vi "Processing Loop.vi"(8 "error in":errorcluster, 11 "Queue in":refnum<queue>) -> (0 "error out":errorcluster)   [LabVIEW 2013, in "LVTM.lvlib"]
uses:
  LVTM.lvlib
  Controls_LVTM/SharedDataDVR.ctl
  Plugin/LVTM_Plugin.lvclass
  Controls_LVTM/LVTM_Config_Info.ctl
  Controls_LVTM/View.ctl
  TCP_Server/TCP_Server.lvclass
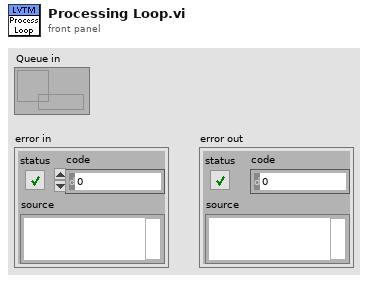
[diagram p1: front panel]
types:
  T1 = typedef "LVTM.lvlib/LVTM_Config_Info.ctl" = cluster{"Data Tree Ref":refnum<vi>, "FP Ref":refnum<vi>, "Column Data Type":enum16{"String", "Numeric"}[], "Search Clones Up To":i32, "SortOptions":cluster{"Col.pri":i32, "RevDir.pri":bool, "Col.sec":i32, "RevDir.sec":bool}, "Group/Flat (0:group)":bool, "CollapsedNodes":string[], "Show/Hide Cols":bool[], "Filtered Paths":path[], "View":T2, "File Extension Filters":string[], "Filter Global VIs":bool, "Shared":refnum<data-value>, "Active Filters":refnum<vi>, "Refresh Rate (ms)":i32, "App Instance Ring Ref":refnum<vi>, "Processing Q":refnum<queue>, "VI Ref":refnum<vi>}
  T2 = typedef "LVTM.lvlib/View.ctl" = enum16{"Group By Library", "Group By Folder", "Flat List"}
  T3 = cluster{"Shared":refnum<data-value>, "Plugins":refnum<class "LVTM_Plugin.lvclass">[], "UIConfig":T1}
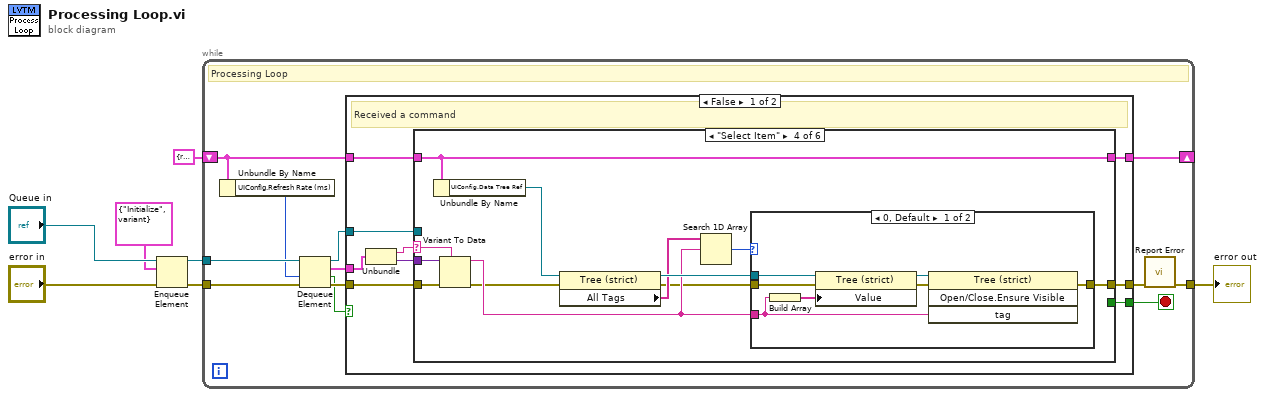
[diagram p0: block diagram]
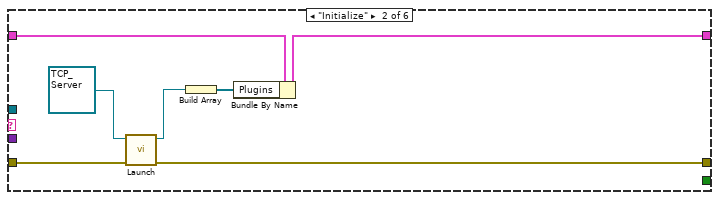
[diagram p3: hidden frame]
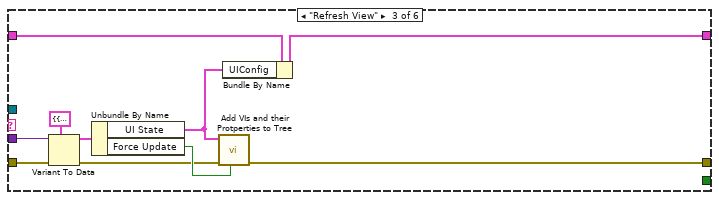
[diagram p4: hidden frame]
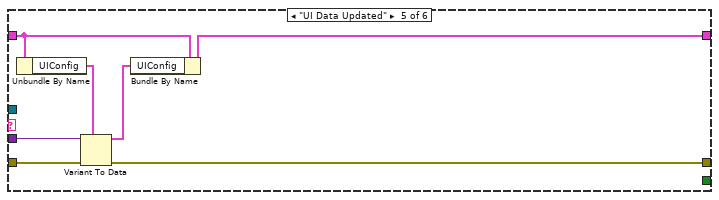
[diagram p6: hidden frame]
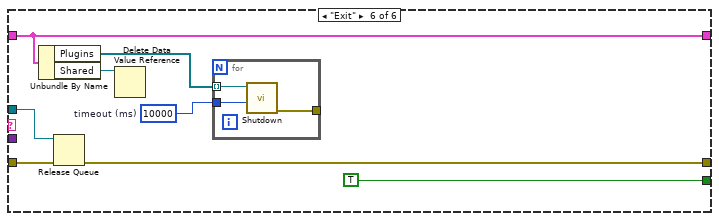
[diagram p7: hidden frame]
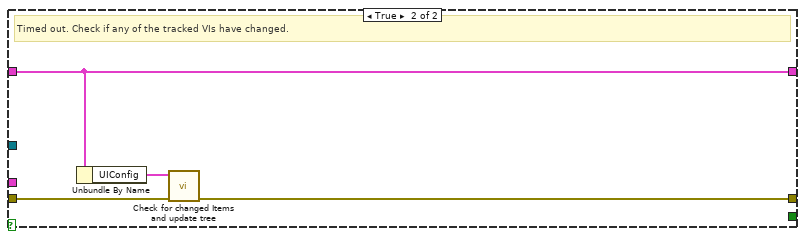
[diagram p8: hidden frame]
diagram:
  n1 = Enqueue Element(queue="Queue in", element=cluster{"Command":string, "Data":variant} {"Command"="Initialize", "Data"=variant}, error in (no error)="error in") -> (queue out=w3:refnum<queue>, error out=w5:errorcluster)  [unwired: 1 in, 1 out]
  n2 = while {
    tunnel: w5 -> [w17]
    shift-right: [w19] -> _
    shift-left: T3 {"Shared"=refnum, "Plugins"=[], "UIConfig"={"Data Tree Ref"=refnum, "FP Ref"=refnum, "Column Data Type"=[], "Search Clones Up To"=100, "SortOptions"={"Col.pri"=0, "RevDir.pri"=FALSE, "Col.sec"=0, "RevDir.sec"=FALSE}, "Group/Flat (0:group)"=FALSE, "CollapsedNodes"=[], "Show/Hide Cols"=[], "Filtered Paths"=[], "View"=enum."Group By Library", "File Extension Filters"=[], "Filter Global VIs"=FALSE, "Shared"=refnum, "Active Filters"=refnum, "Refresh Rate (ms)"=0, "App Instance Ring Ref"=refnum, "Processing Q"=refnum, "VI Ref"=refnum}} -> [w9]
    tunnel: w3 -> [w18]
    tunnel: [w10] -> w6
    stop <- w12 stop-if-true
    # "Processing Loop"
    n3 = Unbundle By Name(w9) -> ("UIConfig.Refresh Rate (ms)"=w8:i32)
    n4 = Dequeue Element(queue=w18, timeout in ms (-1)=w8, error in (no error)=w17) -> (queue out=w11:refnum<queue>, element=w14:cluster{"Command":string, "Data":variant}, timed out?=w15:bool, error out=w16:errorcluster)
    n5 = case shown="False" w15 {
      tunnel: w9 -> [w25 w89]
      tunnel: w16 -> [w22 w87]
      tunnel: [w26 w89] -> w19
      tunnel: [w23 w86] -> w13
      tunnel: w14 -> [w28 _]
      tunnel: [w21 _] -> w12
      tunnel: w11 -> [w20 _]
      frame False {
        # "Received a command"
        n6 = Unbundle(w28) -> ("Command"=w27:string, "Data"=w24:variant)
        n7 = case shown="\"Select Item\"" w27 {
          selector: w27 -> [_ _ _ w57 _ _]
          tunnel: [w30 w35 w39 w56 w72 w78] -> w26
          tunnel: w25 -> [w30 w37 w47 w56 w69 w78]
          tunnel: w24 -> [_ _ w46 w59 w74 _]
          tunnel: [w29 w33 w41 w48 w71 w80] -> w23
          tunnel: w22 -> [w29 w34 w45 w58 w73 w79]
          tunnel: [_ _ _ _ _ TRUE] -> w21
          tunnel: w20 -> [_ _ _ _ _ w81]
          frame "", Default {
          }
          frame "Initialize" {
            n8 = call-dynamic "Launch.vi"("error in (no error)"=w34, "TCP_Server in"=refnum<class "TCP_Server.lvclass"> refnum) -> ("error out"=w33:errorcluster, "TCP_Server out"=w32:refnum<class "TCP_Server.lvclass">)  [unwired: 8 in]
            n9 = Build Array(w32) -> (w31:refnum<class "TCP_Server.lvclass">[])
            n10 = Bundle By Name(cluster=w37, "Plugins"=w31) -> (w35:T3)
          }
          frame "Refresh View" {
            n11 = Variant To Data(error in=w45, type=cluster{"UI State":T1, "Force Update":bool} {"UI State"={"Data Tree Ref"=refnum, "FP Ref"=refnum, "Column Data Type"=[], "Search Clones Up To"=0, "SortOptions"={"Col.pri"=0, "RevDir.pri"=FALSE, "Col.sec"=0, "RevDir.sec"=FALSE}, "Group/Flat (0:group)"=FALSE, "CollapsedNodes"=[], "Show/Hide Cols"=[], "Filtered Paths"=[], "View"=enum."Group By Library", "File Extension Filters"=[], "Filter Global VIs"=FALSE, "Shared"=refnum, "Active Filters"=refnum, "Refresh Rate (ms)"=0, "App Instance Ring Ref"=refnum, "Processing Q"=refnum, "VI Ref"=refnum}, "Force Update"=FALSE}, Variant=w46) -> (data=w44:cluster{"UI State":T1, "Force Update":bool}, error out=w40:errorcluster)
            n12 = Unbundle By Name(w44) -> ("UI State"=w38:T1, "Force Update"=w42:bool)
            n13 = call "Add VIs and their Protperties to Tree.vi"("Force Tree Update (F)"=w42, "error in"=w40, "ConfigInfo in"=w38) -> ("error out"=w41:errorcluster)  [unwired: 7 in, 1 out]
            n14 = Bundle By Name(cluster=w47, "UIConfig"=w38) -> (w39:T3)
          }
          frame "Select Item" {
            n15 = Unbundle By Name(w56) -> ("UIConfig.Data Tree Ref"=w55:refnum<vi>)
            n16 = Variant To Data(error in=w58, type=w57, Variant=w59) -> (data=w52:string, error out=w51:errorcluster)
            n17 = property class="Tree (strict)"(reference=w55, error in=w51) -> (reference out=w54:refnum<vi>, error out=w49:errorcluster, "All Tags"=w53:string[])
            n18 = Search 1D Array(1D array=w53, element=w52) -> (index of element=w50:i32)  [unwired: 1 in]
            n19 = case shown="0, Default" w50 {
              tunnel: w54 -> [w65 _]
              tunnel: w52 -> [w63 _]
              tunnel: w49 -> [w64 w67]
              tunnel: [w60 w67] -> w48
              frame 0, Default {
                n20 = Build Array(w63) -> (w66:string[])
                n21 = property class="Tree (strict)"(reference=w65, error in=w64, "Value"=w66) -> (reference out=w62:refnum<vi>, error out=w61:errorcluster)
                n22 = invoke class="Tree (strict)" method="Open/Close.Ensure Visible"(reference=w62, error in=w61, "tag"=w63) -> (error out=w60:errorcluster)  [unwired: 1 in, 3 out]
              }
              frame -1 {
              }
            }
          }
          frame "UI Data Updated" {
            n23 = Unbundle By Name(w69) -> ("UIConfig"=w68:T1)
            n24 = Variant To Data(error in=w73, type=w68, Variant=w74) -> (data=w70:T1, error out=w71:errorcluster)
            n25 = Bundle By Name(cluster=w69, "UIConfig"=w70) -> (w72:T3)
          }
          frame "Exit" {
            w75 = 10000  # timeout (ms)
            n26 = Unbundle By Name(w78) -> ("Plugins"=w76:refnum<class "LVTM_Plugin.lvclass">[], "Shared"=w77:refnum<data-value>)
            n27 = Release Queue(queue=w81, error in (no error)=w79) -> (error out=w80:errorcluster)  [unwired: 1 in, 2 out]
            n28 = Delete Data Value Reference(data value reference=w77) -> ()  [unwired: 1 in, 2 out]
            n29 = for {
              tunnel: w76 -> [w85] mode=indexing
              tunnel: w75 -> [w84]
              tunnel: [w83] -> _
              n30 = call-dynamic "Shutdown.vi"("timeout in ms (-1)"=w84, "LVTM_Plugin"=w85) -> ("error out"=w83:errorcluster)  [unwired: 8 in, 1 out]
            }
          }
        }
      }
      frame True {
        # "Timed out. Check if any of the tracked VIs have changed."
        n31 = Unbundle By Name(w89) -> ("UIConfig"=w88:T1)
        n32 = call "Check for changed Items and update tree.vi"("error in"=w87, "Configuration"=w88) -> ("error out"=w86:errorcluster)  [unwired: 9 in]
      }
    }
    n33 = call "Report Error.vi"("error in"=w13) -> ("error out"=w10:errorcluster)  [unwired: 10 in]
  }
  "error out" <- w6
